vi "LSMcontroller_v65_updatedsealtest.vi"() -> ()   [LabVIEW 2015] (continued)
                                n2111 = property on="upleft" class="Bool (strict)"("Value"=w5072) -> ()  [unwired: 2 in, 2 out]
                                n2112 = property on="upright" class="Bool (strict)"("Value"=w5072) -> ()  [unwired: 2 in, 2 out]
                                n2113 = property on="downleft" class="Bool (strict)"("Value"=w5072) -> ()  [unwired: 2 in, 2 out]
                                n2114 = property on="downright" class="Bool (strict)"("Value"=w5072) -> ()  [unwired: 2 in, 2 out]
                                }
                                }
                                }
                                }
                                }
                              }
                              n2115 = dll-call lib="phlib.dll" fn="_PH_GetCountRate@8" label="PH_GetCountRate"("devidx"=w5019, "channel"=1) -> (→"Ch1Rate":i32)  [unwired: 5 in, 2 out]
                              n2116 = local read "Stop"() -> (w5021:bool)
                              n2117 = local write "points recorded"(w5018) -> ()
                            }
                          }
                          frame #3 {
                            w5081 = FALSE ("Value (Signaling)")
                            n2118 = call "2pparameters.vi"("command"="get") -> ("params out"=w5075:T10)  [unwired: 1 in]
                            n2119 = Unbundle By Name(w5075) -> ("autoshutter"=w5076:bool)
                            n2120 = case shown="True" w5076 {
                              frame False {
                              }
                              frame True {
                                n2121 = call "shuttercontrol.vi"("command"="close") -> ()  [unwired: 1 in, 1 out]
                              }
                            }
                            n2122 = property on="Start" class="Bool (strict)"("Val(Sgnl)"=w5081) -> ()  [unwired: 2 in, 2 out]
                            n2123 = property on="Start" class="Bool (strict)"("Visible"=TRUE, "DisabledEnum"=T7."Enabled" ("Disabled")) -> ()  [unwired: 2 in, 2 out]
                            n2124 = property on="Stop" class="Bool (strict)"("Val(Sgnl)"=w5081) -> ()  [unwired: 2 in, 2 out]
                            n2125 = property on="Stop" class="Bool (strict)"("Visible"=FALSE, "DisabledEnum"=T7."Disabled" ("Disabled")) -> ()  [unwired: 2 in, 2 out]
                          }
                        }
                      }
                      frame Enabled {
                      }
                    }
                    n2126 = local write "64bit disabled"(TRUE ("64bit disabled")) -> ()
                  }
                }
              }
            }
          }
          event "avpp", "Angle ref", "xpixels ref", "Vx-min ref", "Vx-max ref", "ypixels ref", "Vy-min ref", "Vy-max ref", "ROI Type", "Sampling rate": Value Change {
            n2127 = event-data() -> ()  [unwired: 1 in, 6 out]
            n2128 = local read "avpp"() -> (w5100:i32)
            n2129 = local read "Angle ref"() -> (w5099:dbl)
            n2130 = local read "ROI Type"() -> (w5098:u16)
            n2131 = local read "xpixels ref"() -> (w5095:i32)
            n2132 = local read "Vx-min ref"() -> (w5094:dbl)
            n2133 = local read "Vx-max ref"() -> (w5093:dbl)
            n2134 = local read "ypixels ref"() -> (w5091:i32)
            n2135 = local read "Vy-min ref"() -> (w5092:dbl)
            n2136 = local read "Vy-max ref"() -> (w5088:dbl)
            n2137 = local read "Sampling rate"() -> (w5083:dbl)
            n2138 = local read "# of frames"() -> (w5087:i32)
            n2139 = local read "maxbufferAI"() -> (w5086:i32)
            n2140 = local read "Override AI buffer"() -> (w5084:bool)
            n2141 = call "2pparameters.vi"("command"="get") -> ("params out"=w5097:T10)  [unwired: 1 in]
            n2142 = Bundle By Name(cluster=w5097, "avpp"=w5100, "Angle Img"=w5099, "Xpixels Img"=w5095, "Vx-min Img"=w5094, "VX-max Img"=w5093, "Ypixels Img"=w5091, "Vy-min Img"=w5092, "Vy-max Img"=w5088, "srate"=w5083, "srate Img"=w5083, "measpoints"=w5087, "maxbufferAI"=w5086, "Drawing Mode"=w5098, "Vz-reset"=0.0, "AIoverride"=w5084) -> (w5089:T10)
            n2143 = call "2pparameters.vi"("Params in"=w5089, "command"="set") -> ()  [unwired: 1 out]
          }
          event "# of frames": Value Change {
            n2144 = event-data() -> ()  [unwired: 1 in, 6 out]
            n2145 = local read "Meastab"() -> (w5101:enum32{"X-Y Image", "Linescan", "Timetrace"})
            n2146 = case shown="\"X-Y Image\", Default" w5101 {
              frame "X-Y Image", Default {
                n2147 = local read "# of frames"() -> (w5102:i32)
                n2148 = call "2pparameters.vi"("command"="get") -> ("params out"=w5106:T10)  [unwired: 1 in]
                n2149 = Bundle By Name(cluster=w5106, "measpoints"=w5102) -> (w5103:T10)
                n2150 = call "2pparameters.vi"("Params in"=w5103, "command"="set") -> ()  [unwired: 1 out]
              }
              frame "Linescan" {
                n2151 = local read "srateAODOtt"() -> (w5116:dbl)
                n2152 = local read "# of frames"() -> (w5112:i32)
                n2153 = local read "refreshtime"() -> (w5118:dbl)
                n2154 = local read "bin"() -> (w5113:dbl)
                n2155 = call "tt_timeandsamples.vi"("bin"=w5113, "refreshtime"=w5118, "srateAODOtt"=w5116, "tot#ofsamples"=w5112) -> ("refreshrate"=w5115:dbl, "refreshbuffer"=w5114:i32, "timetracecycles"=w5111:i32)  [unwired: 5 in]
                n2156 = call "2pparameters.vi"("command"="get") -> ("params out"=w5108:T10)  [unwired: 1 in]
                n2157 = Bundle By Name(cluster=w5108, "measpoints"=w5112, "tt_cycles"=w5111, "refreshbuffer"=w5114, "refreshrate"=w5115) -> (w5110:T10)
                n2158 = Reciprocal(x=w5115) -> (1/x=w5117:dbl)
                n2159 = local write "refreshtime"(w5117) -> ()
                n2160 = call "2pparameters.vi"("Params in"=w5110, "command"="set") -> ()  [unwired: 1 out]
              }
              frame "Timetrace" {
                n2161 = local read "srateAODOtt"() -> (w5128:dbl)
                n2162 = local read "# of frames"() -> (w5124:i32)
                n2163 = local read "refreshtime"() -> (w5130:dbl)
                n2164 = local read "bin"() -> (w5125:dbl)
                n2165 = call "tt_timeandsamples.vi"("bin"=w5125, "refreshtime"=w5130, "srateAODOtt"=w5128, "tot#ofsamples"=w5124) -> ("refreshrate"=w5127:dbl, "refreshbuffer"=w5126:i32, "timetracecycles"=w5123:i32)  [unwired: 5 in]
                n2166 = call "2pparameters.vi"("command"="get") -> ("params out"=w5120:T10)  [unwired: 1 in]
                n2167 = Bundle By Name(cluster=w5120, "measpoints"=w5124, "tt_cycles"=w5123, "refreshbuffer"=w5126, "refreshrate"=w5127) -> (w5122:T10)
                n2168 = Reciprocal(x=w5127) -> (1/x=w5129:dbl)
                n2169 = local write "refreshtime"(w5129) -> ()
                n2170 = call "2pparameters.vi"("Params in"=w5122, "command"="set") -> ()  [unwired: 1 out]
              }
            }
          }
          event "srateAODOtt", "refreshtime", "Vx-ref", "Vy-ref", "Vx-min draw", "Vx-max draw", "Vy-min draw", "Vy-max draw", "bin": Value Change {
            n2171 = event-data() -> ()  [unwired: 1 in, 6 out]
            n2172 = local read "ypixels ref"() -> (w5162:i32)
            n2173 = local read "Vy-min draw"() -> (w5138:dbl)
            n2174 = local read "Vy-max draw"() -> (w5137:dbl)
            n2175 = local read "Vx-min draw"() -> (w5140:dbl)
            n2176 = local read "Vx-max draw"() -> (w5139:dbl)
            n2177 = local read "xpixels ref"() -> (w5136:i32)
            n2178 = local read "ROI Type"() -> (w5135:u16)
            n2179 = local read "Pel"() -> (w5134:dbl)
            n2180 = local read "srateAODOtt"() -> (w5144:dbl)
            n2181 = local read "# of frames"() -> (w5149:i32)
            n2182 = local read "refreshtime"() -> (w5142:dbl)
            n2183 = local read "bin"() -> (w5147:dbl)
            n2184 = local read "Override AI buffer"() -> (w5132:bool)
            n2185 = local read "finite samples"() -> (w5156:bool)
            n2186 = local read "srateAODOtt"() -> (w5131:dbl)
            n2187 = local read "srateAODOtt"() -> (w5150:dbl)
            n2188 = local read "continuous"() -> (w5155:bool)
            n2189 = local read "Angle ref"() -> (w5141:dbl)
            n2190 = local read "wavdet"() -> (w5157:bool)
            n2191 = local read "Vx-ref"() -> (w5152:dbl)
            n2192 = local read "Vy-ref"() -> (w5154:dbl)
            n2193 = local read "avpp"() -> (w5153:i32)
            n2194 = call "tt_timeandsamples.vi"("bin"=w5147, "refreshtime"=w5142, "srateAODOtt"=w5144, "tot#ofsamples"=w5149) -> ("refreshrate"=w5145:dbl, "refreshbuffer"=w5146:i32, "timetracecycles"=w5151:i32)  [unwired: 5 in]
            n2195 = local read "bin"() -> (w5148:dbl)
            n2196 = call "2pparameters.vi"("command"="get") -> ("params out"=w5160:T10)  [unwired: 1 in]
            n2197 = Bundle By Name(cluster=w5160, "Drawing Mode"=w5135, "measpoints"=w5149, "tt_cycles"=w5151, "refreshbuffer"=w5146, "refreshrate"=w5145, "Vx-ref"=w5152, "Vy-ref"=w5154, "srate"=w5131, "finite"=w5156, "cont"=w5155, "wavdet"=w5157, "avpp"=w5153, "srateAODO"=w5150, "bufferAI"=w5146, "bin"=w5148, "Angle Img"=w5141, "Vxminref"=w5140, "Vxmaxref"=w5139, "Vyminref"=w5138, "Vymaxref"=w5137, "Xpixels Img"=w5136, "Ypixels Img"=w5162, "Pel"=w5134, "Vz-reset"=0.0, "AIoverride"=w5132) -> (w5158:T10)
            n2198 = Reciprocal(x=w5145) -> (1/x=w5143:dbl)
            n2199 = local write "refreshtime"(w5143) -> ()
            n2200 = call "2pparameters.vi"("Params in"=w5158, "command"="set") -> ()  [unwired: 1 out]
          }
          event "Init": Value Change {
            # "Disabled for conversion to 64 bit"
            n2201 = event-data() -> ()  [unwired: 1 in, 6 out]
            n2202 = disable-structure shown="Disabled" {
              frame Disabled {
                n2203 = flat-sequence {
                  frame #0 {
                    n2204 = local read "Measurement"() -> (w5164:T4)
                    n2205 = case shown="\"Lifetime (scan)\", \"Lifetime (contour)\"" w5164 {
                      frame "X-Y-t movie", Default {
                      }
                      frame "Lifetime (point)" {
                        n2206 = stacked-sequence {
                          frame #0 {
                            n2207 = call "initialize.vi"("mode"=0) -> ()
                          }
                          frame #1 {
                            n2208 = call "calib.vi"() -> ()  [unwired: 1 in]
                          }
                        }
                      }
                      frame "Lifetime (scan)", "Lifetime (contour)" {
                        n2209 = stacked-sequence {
                          frame #0 {
                            n2210 = call "initialize.vi"("mode"=3) -> ()
                          }
                          frame #1 {
                            n2211 = call "calib.vi"() -> ()  [unwired: 1 in]
                          }
                        }
                      }
                    }
                  }
                  frame #1 {
                    n2212 = property on="Start" class="Bool (strict)"("Visible"=TRUE, "DisabledEnum"=T7."Enabled" ("Disabled")) -> ()  [unwired: 2 in, 2 out]
                    n2213 = property on="Init" class="Bool (strict)"("Visible"=FALSE, "DisabledEnum"=T7."Disabled and Grayed Out" ("Disabled"), "Value"=FALSE ("Init")) -> ()  [unwired: 2 in, 2 out]
                  }
                }
              }
              frame Enabled {
              }
            }
            n2214 = local write "64bit disabled"(TRUE ("64bit disabled")) -> ()
          }
          event "Measurement": Value Change {
            n2215 = event-data() -> ()  [unwired: 1 in, 5 out]
            n2216 = case shown="\"Lifetime (scan)\"" "Measurement" {
              frame "X-Y-t movie" {
                w5179 = T7."Disabled" ("Disabled")
                w5178 = FALSE ("Visible")
                n2217 = call "2pparameters.vi"("command"="get") -> ("params out"=w5189:T10)  [unwired: 1 in]
                n2218 = local write "graphtab"(T5."image" ("graphtab")) -> ()
                n2219 = local write "Save tab"(enum32{"withsave", "withoutsave"}."withsave" ("Save tab")) -> ()
                n2220 = Bundle By Name(cluster=w5189, "type"="X-Y-t movie") -> (w5187:T10)
                n2221 = call "2pparameters.vi"("Params in"=w5187, "command"="set") -> ()  [unwired: 1 out]
                n2222 = property on="refreshtime" class="DigNum (strict)"("Visible"=FALSE, "DisabledEnum"=T7."Disabled and Grayed Out" ("Disabled")) -> ()  [unwired: 2 in, 2 out]
                n2223 = property on="Start" class="Bool (strict)"("Visible"=TRUE, "DisabledEnum"=T7."Enabled" ("Disabled")) -> ()  [unwired: 2 in, 2 out]
                n2224 = property on="Init" class="Bool (strict)"("Visible"=FALSE, "DisabledEnum"=T7."Disabled and Grayed Out" ("Disabled"), "Value"=FALSE ("Init")) -> ()  [unwired: 2 in, 2 out]
                n2225 = property on="ttt" class="Enum (strict)"("Visible"=FALSE) -> ()  [unwired: 2 in, 2 out]
                n2226 = property on="# of frames" class="DigNum (strict)"("DisabledEnum"=T7."Enabled" ("Disabled"), "Caption.Text"="# of frames") -> ()  [unwired: 2 in, 2 out]
                n2227 = property on="continuous" class="Bool (strict)"("Visible"=TRUE, "DisabledEnum"=T7."Enabled" ("Disabled")) -> ()  [unwired: 2 in, 2 out]
                n2228 = property on="finite samples" class="Bool (strict)"("Visible"=TRUE, "DisabledEnum"=T7."Enabled" ("Disabled")) -> ()  [unwired: 2 in, 2 out]
                n2229 = property on="avpp" class="DigNum (strict)"("Visible"=TRUE, "DisabledEnum"=T7."Enabled" ("Disabled")) -> ()  [unwired: 2 in, 2 out]
                n2230 = property on="srateAODOtt" class="DigNum (strict)"("Visible"=FALSE, "DisabledEnum"=T7."Disabled" ("Disabled")) -> ()  [unwired: 2 in, 2 out]
                n2231 = local write "save\ndata"(TRUE ("save\ndata")) -> ()
                n2232 = property on="finite samples" class="Bool (strict)"("Val(Sgnl)"=TRUE ("continuous for display")) -> ()  [unwired: 2 in, 2 out]
                n2233 = property on="continuous" class="Bool (strict)"("Value"=FALSE ("continuous for display")) -> ()  [unwired: 2 in, 2 out]
                n2234 = property on="Current Average" class="DigNum (strict)"("Visible"=TRUE, "DisabledEnum"=T7."Enabled" ("Disabled")) -> ()  [unwired: 2 in, 2 out]
                n2235 = property on="img_CH1" class="IntGraph (strict)"("ZScale.Maximum"=7.0 ("Z Scale.Range:Maximum")) -> ()  [unwired: 2 in, 2 out]
                n2236 = property on="Sampling rate" class="DigNum (strict)"("Visible"=TRUE, "DisabledEnum"=T7."Enabled" ("Disabled")) -> ()  [unwired: 2 in, 2 out]
                n2237 = property on="Pel" class="DigNum (strict)"("Visible"=w5178, "DisabledEnum"=w5179) -> ()  [unwired: 2 in, 2 out]
                n2238 = property on="bin" class="DigNum (strict)"("Visible"=w5178, "DisabledEnum"=w5179) -> ()  [unwired: 2 in, 2 out]
                "Meastab" <- enum32{"X-Y Image", "Linescan", "Timetrace"}."X-Y Image" ("Meastab")
                "Zscantab" <- enum32{"withzscan", "withoutzscan", "lifetime"}."withoutzscan" ("Zscantab")
              }
              frame "X-Y-Z stack" {
                w5216 = T7."Disabled" ("Disabled")
                w5215 = FALSE ("Visible")
                n2239 = call "2pparameters.vi"("command"="get") -> ("params out"=w5226:T10)  [unwired: 1 in]
                n2240 = call "2pparameters.vi"("command"="get") -> ("params out"=w5230:T10)  [unwired: 1 in]
                n2241 = Bundle By Name(cluster=w5226, "type"="X-Y-Z stack") -> (w5224:T10)
                n2242 = Unbundle By Name(w5230) -> ("motorref"=w5229:refnum<k7>)
                n2243 = call "2pparameters.vi"("Params in"=w5224, "command"="set") -> ()  [unwired: 1 out]
                n2244 = local write "Zscantab"(enum32{"withzscan", "withoutzscan", "lifetime"}."withzscan" ("Zscantab")) -> ()
                n2245 = local write "Meastab"(enum32{"X-Y Image", "Linescan", "Timetrace"}."X-Y Image" ("Meastab")) -> ()
                n2246 = invoke class="MG17Motor" method="GetPosition"(reference=w5229, "lChanID"=0, "pfPosition"=sgl 0.0) -> ("pfPosition"=w5241:sgl)  [unwired: 2 in, 4 out]
                n2247 = property on="refreshtime" class="DigNum (strict)"("Visible"=FALSE, "DisabledEnum"=T7."Disabled and Grayed Out" ("Disabled")) -> ()  [unwired: 2 in, 2 out]
                n2248 = property on="Start" class="Bool (strict)"("Visible"=TRUE, "DisabledEnum"=T7."Enabled" ("Disabled")) -> ()  [unwired: 2 in, 2 out]
                n2249 = property on="Init" class="Bool (strict)"("Visible"=FALSE, "DisabledEnum"=T7."Disabled and Grayed Out" ("Disabled"), "Value"=FALSE ("Init")) -> ()  [unwired: 2 in, 2 out]
                n2250 = property on="ttt" class="Enum (strict)"("Visible"=FALSE) -> ()  [unwired: 2 in, 2 out]
                n2251 = Multiply(x=w5241, y=1000.0) -> (x*y=w5240:dbl)
                n2252 = local write "Actual Z position"(w5240) -> ()
                n2253 = local write "Save tab"(enum32{"withsave", "withoutsave"}."withsave" ("Save tab")) -> ()
                n2254 = property on="finite samples" class="Bool (strict)"("Visible"=FALSE, "DisabledEnum"=T7."Disabled and Grayed Out" ("Disabled")) -> ()  [unwired: 2 in, 2 out]
                n2255 = property on="avpp" class="DigNum (strict)"("Visible"=TRUE, "DisabledEnum"=T7."Enabled" ("Disabled")) -> ()  [unwired: 2 in, 2 out]
                n2256 = property on="continuous" class="Bool (strict)"("Visible"=FALSE, "DisabledEnum"=T7."Disabled and Grayed Out" ("Disabled")) -> ()  [unwired: 2 in, 2 out]
                n2257 = property on="img_CH1" class="IntGraph (strict)"("ZScale.Maximum"=7.0 ("Z Scale.Range:Maximum")) -> ()  [unwired: 2 in, 2 out]
                n2258 = property on="srateAODOtt" class="DigNum (strict)"("Visible"=FALSE, "DisabledEnum"=T7."Disabled" ("Disabled")) -> ()  [unwired: 2 in, 2 out]
                n2259 = property on="Pel" class="DigNum (strict)"("Visible"=w5215, "DisabledEnum"=w5216) -> ()  [unwired: 2 in, 2 out]
                n2260 = property on="bin" class="DigNum (strict)"("Visible"=w5215, "DisabledEnum"=w5216) -> ()  [unwired: 2 in, 2 out]
                n2261 = property on="Current Average" class="DigNum (strict)"("Visible"=TRUE, "DisabledEnum"=T7."Enabled" ("Disabled")) -> ()  [unwired: 2 in, 2 out]
                n2262 = property on="# of frames" class="DigNum (strict)"("Caption.Text"="# of slices", "DisabledEnum"=T7."Disabled and Grayed Out" ("Disabled")) -> ()  [unwired: 2 in, 2 out]
                n2263 = local write "save\ndata"(TRUE ("save\ndata")) -> ()
                n2264 = property on="finite samples" class="Bool (strict)"("Val(Sgnl)"=TRUE ("continuous for display")) -> ()  [unwired: 2 in, 2 out]
                n2265 = property on="continuous" class="Bool (strict)"("Value"=FALSE ("continuous for display")) -> ()  [unwired: 2 in, 2 out]
                n2266 = property on="Sampling rate" class="DigNum (strict)"("Visible"=TRUE, "DisabledEnum"=T7."Enabled" ("Disabled")) -> ()  [unwired: 2 in, 2 out]
              }
              frame "X-Y-Z-t movie" {
                w5260 = T7."Disabled" ("Disabled")
                w5259 = FALSE ("Visible")
                n2267 = property on="# of frames" class="DigNum (strict)"("DisabledEnum"=T7."Enabled" ("Disabled")) -> ()  [unwired: 2 in, 2 out]
                n2268 = property on="Current Average" class="DigNum (strict)"("Visible"=TRUE, "DisabledEnum"=T7."Enabled" ("Disabled")) -> ()  [unwired: 2 in, 2 out]
                n2269 = property on="avpp" class="DigNum (strict)"("Visible"=TRUE, "DisabledEnum"=T7."Enabled" ("Disabled")) -> ()  [unwired: 2 in, 2 out]
                n2270 = local write "Save tab"(enum32{"withsave", "withoutsave"}."withsave" ("Save tab")) -> ()
                n2271 = local write "Zscantab"(enum32{"withzscan", "withoutzscan", "lifetime"}."withzscan" ("Zscantab")) -> ()
                n2272 = local write "Meastab"(enum32{"X-Y Image", "Linescan", "Timetrace"}."X-Y Image" ("Meastab")) -> ()
                n2273 = property on="Start" class="Bool (strict)"("Visible"=TRUE, "DisabledEnum"=T7."Enabled" ("Disabled")) -> ()  [unwired: 2 in, 2 out]
                n2274 = property on="refreshtime" class="DigNum (strict)"("Visible"=FALSE, "DisabledEnum"=T7."Disabled and Grayed Out" ("Disabled")) -> ()  [unwired: 2 in, 2 out]
                n2275 = property on="Init" class="Bool (strict)"("Visible"=FALSE, "DisabledEnum"=T7."Disabled and Grayed Out" ("Disabled"), "Value"=FALSE ("Init")) -> ()  [unwired: 2 in, 2 out]
                n2276 = property on="ttt" class="Enum (strict)"("Visible"=FALSE) -> ()  [unwired: 2 in, 2 out]
                n2277 = call "2pparameters.vi"("command"="get") -> ("params out"=w5270:T10)  [unwired: 1 in]
                n2278 = Bundle By Name(cluster=w5270, "type"="X-Y-Z-t movie") -> (w5268:T10)
                n2279 = property on="continuous" class="Bool (strict)"("Visible"=TRUE, "DisabledEnum"=T7."Enabled" ("Disabled")) -> ()  [unwired: 2 in, 2 out]
                n2280 = property on="finite samples" class="Bool (strict)"("Visible"=TRUE, "DisabledEnum"=T7."Enabled" ("Disabled")) -> ()  [unwired: 2 in, 2 out]
                n2281 = call "2pparameters.vi"("Params in"=w5268, "command"="set") -> ()  [unwired: 1 out]
                n2282 = property on="srateAODOtt" class="DigNum (strict)"("Visible"=FALSE, "DisabledEnum"=T7."Disabled" ("Disabled")) -> ()  [unwired: 2 in, 2 out]
                n2283 = local write "save\ndata"(TRUE ("save\ndata")) -> ()
                n2284 = property on="img_CH1" class="IntGraph (strict)"("ZScale.Maximum"=7.0 ("Z Scale.Range:Maximum")) -> ()  [unwired: 2 in, 2 out]
                n2285 = property on="continuous" class="Bool (strict)"("Value"=FALSE ("continuous for display")) -> ()  [unwired: 2 in, 2 out]
                n2286 = property on="finite samples" class="Bool (strict)"("Value"=TRUE ("continuous for display")) -> ()  [unwired: 2 in, 2 out]
                n2287 = property on="Sampling rate" class="DigNum (strict)"("Visible"=TRUE, "DisabledEnum"=T7."Enabled" ("Disabled")) -> ()  [unwired: 2 in, 2 out]
                n2288 = property on="Pel" class="DigNum (strict)"("Visible"=w5259, "DisabledEnum"=w5260) -> ()  [unwired: 2 in, 2 out]
                n2289 = property on="bin" class="DigNum (strict)"("Visible"=w5259, "DisabledEnum"=w5260) -> ()  [unwired: 2 in, 2 out]
              }
              frame "linescan" {
                w5295 = T7."Enabled" ("Disabled")
                w5294 = TRUE ("Visible")
                w5297 = T7."Enabled" ("Disabled")
                w5296 = TRUE ("Visible")
                n2290 = local write "Meastab"(enum32{"X-Y Image", "Linescan", "Timetrace"}."Linescan" ("Meastab")) -> ()
                n2291 = property on="Current Average" class="DigNum (strict)"("Visible"=TRUE, "DisabledEnum"=T7."Enabled" ("Disabled")) -> ()  [unwired: 2 in, 2 out]
                n2292 = property on="ttt" class="Enum (strict)"("Visible"=FALSE) -> ()  [unwired: 2 in, 2 out]
                n2293 = local write "Save tab"(enum32{"withsave", "withoutsave"}."withsave" ("Save tab")) -> ()
                n2294 = local write "Zscantab"(enum32{"withzscan", "withoutzscan", "lifetime"}."withoutzscan" ("Zscantab")) -> ()
                n2295 = property on="refreshtime" class="DigNum (strict)"("Visible"=FALSE, "DisabledEnum"=T7."Disabled and Grayed Out" ("Disabled")) -> ()  [unwired: 2 in, 2 out]
                n2296 = property on="continuous" class="Bool (strict)"("Value"=FALSE ("continuous for display")) -> ()  [unwired: 2 in, 2 out]
                n2297 = property on="finite samples" class="Bool (strict)"("Value"=TRUE ("continuous for display")) -> ()  [unwired: 2 in, 2 out]
                n2298 = local write "save\ndata"(TRUE ("save\ndata")) -> ()
                n2299 = property on="Start" class="Bool (strict)"("Visible"=TRUE, "DisabledEnum"=T7."Enabled" ("Disabled")) -> ()  [unwired: 2 in, 2 out]
                n2300 = property on="Init" class="Bool (strict)"("Visible"=FALSE, "DisabledEnum"=T7."Disabled and Grayed Out" ("Disabled"), "Value"=FALSE ("Init")) -> ()  [unwired: 2 in, 2 out]
                n2301 = call "2pparameters.vi"("command"="get") -> ("params out"=w5306:T10)  [unwired: 1 in]
                n2302 = Bundle By Name(cluster=w5306, "type"="linescan") -> (w5304:T10)
                n2303 = property on="# of frames" class="DigNum (strict)"("DisabledEnum"=T7."Enabled" ("Disabled"), "Caption.Text"="# of lines") -> ()  [unwired: 2 in, 2 out]
                n2304 = property on="continuous" class="Bool (strict)"("Visible"=TRUE, "DisabledEnum"=T7."Enabled" ("Disabled")) -> ()  [unwired: 2 in, 2 out]
                n2305 = property on="avpp" class="DigNum (strict)"("Visible"=TRUE, "DisabledEnum"=T7."Enabled" ("Disabled")) -> ()  [unwired: 2 in, 2 out]
                n2306 = property on="finite samples" class="Bool (strict)"("Visible"=TRUE, "DisabledEnum"=T7."Enabled" ("Disabled")) -> ()  [unwired: 2 in, 2 out]
                n2307 = property on="srateAODOtt" class="DigNum (strict)"("Visible"=TRUE, "DisabledEnum"=T7."Enabled" ("Disabled")) -> ()  [unwired: 2 in, 2 out]
                n2308 = call "2pparameters.vi"("Params in"=w5304, "command"="set") -> ()  [unwired: 1 out]
                n2309 = property on="Pel" class="DigNum (strict)"("Visible"=w5296, "DisabledEnum"=w5297) -> ()  [unwired: 2 in, 2 out]
                n2310 = property on="bin" class="DigNum (strict)"("Visible"=w5296, "DisabledEnum"=w5297) -> ()  [unwired: 2 in, 2 out]
                n2311 = property on="Sampling rate" class="DigNum (strict)"("Visible"=FALSE, "DisabledEnum"=T7."Disabled" ("Disabled")) -> ()  [unwired: 2 in, 2 out]
                n2312 = property on="Pel" class="DigNum (strict)"("Visible"=w5294, "DisabledEnum"=w5295) -> ()  [unwired: 2 in, 2 out]
                n2313 = property on="bin" class="DigNum (strict)"("Visible"=w5294, "DisabledEnum"=w5295) -> ()  [unwired: 2 in, 2 out]
              }
              frame "Timetrace" {
                w5332 = T7."Enabled" ("Disabled")
                w5331 = TRUE ("Visible")
                n2314 = call "2pparameters.vi"("command"="get") -> ("params out"=w5337:T10)  [unwired: 1 in]
                n2315 = local write "Meastab"(enum32{"X-Y Image", "Linescan", "Timetrace"}."Timetrace" ("Meastab")) -> ()
                n2316 = Unbundle By Name(w5337) -> ("Angle draw"=w5339:dbl)
                n2317 = local write "Zscantab"(enum32{"withzscan", "withoutzscan", "lifetime"}."withoutzscan" ("Zscantab")) -> ()
                n2318 = property on="# of frames" class="DigNum (strict)"("DisabledEnum"=T7."Enabled" ("Disabled"), "Caption.Text"="# of samples") -> ()  [unwired: 2 in, 2 out]
                n2319 = property on="refreshtime" class="DigNum (strict)"("Visible"=TRUE, "DisabledEnum"=T7."Enabled" ("Disabled")) -> ()  [unwired: 2 in, 2 out]
                n2320 = property on="avpp" class="DigNum (strict)"("Visible"=FALSE, "DisabledEnum"=T7."Disabled and Grayed Out" ("Disabled")) -> ()  [unwired: 2 in, 2 out]
                n2321 = property on="Current Average" class="DigNum (strict)"("Visible"=FALSE, "DisabledEnum"=T7."Disabled and Grayed Out" ("Disabled")) -> ()  [unwired: 2 in, 2 out]
                n2322 = local write "Angle drawing"(w5339) -> ()
                n2323 = property on="ttt" class="Enum (strict)"("Visible"=TRUE) -> ()  [unwired: 2 in, 2 out]
                n2324 = property on="continuous" class="Bool (strict)"("Visible"=TRUE, "DisabledEnum"=T7."Enabled" ("Disabled")) -> ()  [unwired: 2 in, 2 out]
                n2325 = property on="finite samples" class="Bool (strict)"("Visible"=TRUE, "DisabledEnum"=T7."Enabled" ("Disabled")) -> ()  [unwired: 2 in, 2 out]
                n2326 = local write "save\ndata"(TRUE ("save\ndata")) -> ()
                n2327 = property on="finite samples" class="Bool (strict)"("Val(Sgnl)"=TRUE ("continuous for display")) -> ()  [unwired: 2 in, 2 out]
                n2328 = property on="continuous" class="Bool (strict)"("Value"=FALSE ("continuous for display")) -> ()  [unwired: 2 in, 2 out]
                n2329 = local write "Save tab"(enum32{"withsave", "withoutsave"}."withsave" ("Save tab")) -> ()
                n2330 = property on="srateAODOtt" class="DigNum (strict)"("Visible"=TRUE, "DisabledEnum"=T7."Enabled" ("Disabled")) -> ()  [unwired: 2 in, 2 out]
                n2331 = call "2pparameters.vi"("command"="get") -> ("params out"=w5344:T10)  [unwired: 1 in]
                n2332 = property on="Start" class="Bool (strict)"("Visible"=TRUE, "DisabledEnum"=T7."Enabled" ("Disabled")) -> ()  [unwired: 2 in, 2 out]
                n2333 = property on="Init" class="Bool (strict)"("Visible"=FALSE, "DisabledEnum"=T7."Disabled and Grayed Out" ("Disabled"), "Value"=FALSE ("Init")) -> ()  [unwired: 2 in, 2 out]
                n2334 = Bundle By Name(cluster=w5344, "type"="Timetrace") -> (w5342:T10)
                n2335 = property on="Sampling rate" class="DigNum (strict)"("Visible"=FALSE, "DisabledEnum"=T7."Disabled" ("Disabled")) -> ()  [unwired: 2 in, 2 out]
                n2336 = property on="Pel" class="DigNum (strict)"("Visible"=w5331, "DisabledEnum"=w5332) -> ()  [unwired: 2 in, 2 out]
                n2337 = property on="bin" class="DigNum (strict)"("Visible"=w5331, "DisabledEnum"=w5332) -> ()  [unwired: 2 in, 2 out]
                n2338 = call "2pparameters.vi"("Params in"=w5342, "command"="set") -> ()  [unwired: 1 out]
              }
              frame "Lifetime (point)" {
                w5365 = T7."Enabled" ("Disabled")
                w5364 = TRUE ("Visible")
                n2339 = property on="Pel" class="DigNum (strict)"("Visible"=w5364, "DisabledEnum"=w5365) -> ()  [unwired: 2 in, 2 out]
                n2340 = property on="bin" class="DigNum (strict)"("Visible"=w5364, "DisabledEnum"=w5365) -> ()  [unwired: 2 in, 2 out]
                n2341 = property on="ttt" class="Enum (strict)"("Visible"=FALSE) -> ()  [unwired: 2 in, 2 out]
                n2342 = local write "Zscantab"(enum32{"withzscan", "withoutzscan", "lifetime"}."lifetime" ("Zscantab")) -> ()
                n2343 = local write "graphtab"(T5."Lifetime" ("graphtab")) -> ()
                n2344 = local write "Meastab"(enum32{"X-Y Image", "Linescan", "Timetrace"}."Timetrace" ("Meastab")) -> ()
                n2345 = call "lifetimeparameters.vi"("command"="get") -> ("Params out"=w5372:T19)  [unwired: 1 in]
                n2346 = Unbundle By Name(w5372) -> ("initialized"=w5373:bool)
                n2347 = property on="srateAODOtt" class="DigNum (strict)"("Visible"=TRUE, "DisabledEnum"=T7."Enabled" ("Disabled")) -> ()  [unwired: 2 in, 2 out]
                n2348 = case shown="False" w5373 {
                  frame False {
                    n2349 = property on="Init" class="Bool (strict)"("Visible"=TRUE, "DisabledEnum"=T7."Enabled" ("Disabled")) -> ()  [unwired: 2 in, 2 out]
                    n2350 = property on="Start" class="Bool (strict)"("Visible"=FALSE, "DisabledEnum"=T7."Disabled and Grayed Out" ("Disabled")) -> ()  [unwired: 2 in, 2 out]
                  }
                  frame True {
                  }
                }
                n2351 = property on="Sampling rate" class="DigNum (strict)"("Visible"=FALSE, "DisabledEnum"=T7."Disabled" ("Disabled")) -> ()  [unwired: 2 in, 2 out]
              }
              frame "Lifetime (scan)" {
                w5382 = T7."Disabled" ("Disabled")
                w5381 = FALSE ("Visible")
                n2352 = call "lifetimeparameters.vi"("command"="get") -> ("Params out"=w5394:T19)  [unwired: 1 in]
                n2353 = local write "graphtab"(T5."image" ("graphtab")) -> ()
                n2354 = local write "Save tab"(enum32{"withsave", "withoutsave"}."withsave" ("Save tab")) -> ()
                n2355 = local write "Meastab"(enum32{"X-Y Image", "Linescan", "Timetrace"}."X-Y Image" ("Meastab")) -> ()
                n2356 = local write "Zscantab"(enum32{"withzscan", "withoutzscan", "lifetime"}."lifetime" ("Zscantab")) -> ()
                n2357 = Unbundle By Name(w5394) -> ("initialized"=w5393:bool)
                n2358 = property on="ttt" class="Enum (strict)"("Visible"=FALSE) -> ()  [unwired: 2 in, 2 out]
                n2359 = property on="refreshtime" class="DigNum (strict)"("Visible"=FALSE, "DisabledEnum"=T7."Disabled and Grayed Out" ("Disabled")) -> ()  [unwired: 2 in, 2 out]
                n2360 = property on="Pel" class="DigNum (strict)"("Visible"=w5381, "DisabledEnum"=w5382) -> ()  [unwired: 2 in, 2 out]
                n2361 = property on="bin" class="DigNum (strict)"("Visible"=w5381, "DisabledEnum"=w5382) -> ()  [unwired: 2 in, 2 out]
                n2362 = property on="save data" class="Bool (strict)"("Visible"=TRUE, "DisabledEnum"=T7."Enabled" ("Disabled"), "Value"=TRUE ("Visible")) -> ()  [unwired: 2 in, 2 out]
                n2363 = case shown="False" w5393 {
                  frame False {
                    n2364 = property on="Init" class="Bool (strict)"("Visible"=TRUE, "DisabledEnum"=T7."Enabled" ("Disabled")) -> ()  [unwired: 2 in, 2 out]
                    n2365 = property on="Start" class="Bool (strict)"("Visible"=FALSE, "DisabledEnum"=T7."Disabled and Grayed Out" ("Disabled")) -> ()  [unwired: 2 in, 2 out]
                  }
                  frame True {
                  }
                }
                n2366 = call "2pparameters.vi"("command"="get") -> ("params out"=w5399:T10)  [unwired: 1 in]
                n2367 = property on="continuous" class="Bool (strict)"("Visible"=TRUE, "DisabledEnum"=T7."Disabled and Grayed Out" ("Disabled")) -> ()  [unwired: 2 in, 2 out]
                n2368 = property on="finite samples" class="Bool (strict)"("Visible"=TRUE, "DisabledEnum"=T7."Enabled" ("Disabled")) -> ()  [unwired: 2 in, 2 out]
                n2369 = Bundle By Name(cluster=w5399, "type"="Lifetime (scan)") -> (w5397:T10)
                n2370 = call "2pparameters.vi"("Params in"=w5397, "command"="set") -> ()  [unwired: 1 out]
                n2371 = property on="finite samples" class="Bool (strict)"("Val(Sgnl)"=TRUE ("continuous for display")) -> ()  [unwired: 2 in, 2 out]
                n2372 = property on="continuous" class="Bool (strict)"("Value"=FALSE ("continuous for display")) -> ()  [unwired: 2 in, 2 out]
                n2373 = property on="srateAODOtt" class="DigNum (strict)"("Visible"=FALSE, "DisabledEnum"=T7."Disabled" ("Disabled")) -> ()  [unwired: 2 in, 2 out]
                n2374 = property on="# of frames" class="DigNum (strict)"("DisabledEnum"=T7."Enabled" ("Disabled"), "Caption.Text"="# of frames") -> ()  [unwired: 2 in, 2 out]
                n2375 = property on="img_CH1" class="IntGraph (strict)"("ZScale.Maximum"=12.5 ("Z Scale.Range:Maximum")) -> ()  [unwired: 2 in, 2 out]
                n2376 = property on="Current Average" class="DigNum (strict)"("Visible"=TRUE, "DisabledEnum"=T7."Enabled" ("Disabled")) -> ()  [unwired: 2 in, 2 out]
                n2377 = property on="Sampling rate" class="DigNum (strict)"("Visible"=TRUE, "DisabledEnum"=T7."Enabled" ("Disabled")) -> ()  [unwired: 2 in, 2 out]
                n2378 = property on="avpp" class="DigNum (strict)"("Visible"=TRUE, "DisabledEnum"=T7."Enabled" ("Disabled")) -> ()  [unwired: 2 in, 2 out]
              }
              frame "Lifetime (contour)" {
                w5423 = T7."Enabled" ("Disabled")
                w5422 = TRUE ("Visible")
                n2379 = call "2pparameters.vi"("command"="get") -> ("params out"=w5430:T10)  [unwired: 1 in]
                n2380 = property on="# of frames" class="DigNum (strict)"("DisabledEnum"=T7."Enabled" ("Disabled"), "Caption.Text"="# of samples") -> ()  [unwired: 2 in, 2 out]
                n2381 = property on="refreshtime" class="DigNum (strict)"("Visible"=TRUE, "DisabledEnum"=T7."Enabled" ("Disabled")) -> ()  [unwired: 2 in, 2 out]
                n2382 = Unbundle By Name(w5430) -> ("Angle draw"=w5432:dbl)
                n2383 = property on="avpp" class="DigNum (strict)"("Visible"=FALSE, "DisabledEnum"=T7."Disabled and Grayed Out" ("Disabled")) -> ()  [unwired: 2 in, 2 out]
                n2384 = property on="Current Average" class="DigNum (strict)"("Visible"=FALSE, "DisabledEnum"=T7."Disabled and Grayed Out" ("Disabled")) -> ()  [unwired: 2 in, 2 out]
                n2385 = local write "Angle drawing"(w5432) -> ()
                n2386 = local write "Save tab"(enum32{"withsave", "withoutsave"}."withsave" ("Save tab")) -> ()
                n2387 = local write "Zscantab"(enum32{"withzscan", "withoutzscan", "lifetime"}."lifetime" ("Zscantab")) -> ()
                n2388 = local write "graphtab"(T5."Lifetime" ("graphtab")) -> ()
                n2389 = local write "Meastab"(enum32{"X-Y Image", "Linescan", "Timetrace"}."Timetrace" ("Meastab")) -> ()
                n2390 = property on="ttt" class="Enum (strict)"("Visible"=TRUE) -> ()  [unwired: 2 in, 2 out]
                n2391 = call "lifetimeparameters.vi"("command"="get") -> ("Params out"=w5454:T19)  [unwired: 1 in]
                n2392 = property on="finite samples" class="Bool (strict)"("Val(Sgnl)"=TRUE ("continuous for display")) -> ()  [unwired: 2 in, 2 out]
                n2393 = local write "save\ndata"(TRUE ("save\ndata")) -> ()
                n2394 = Unbundle By Name(w5454) -> ("initialized"=w5455:bool)
                n2395 = property on="continuous" class="Bool (strict)"("Visible"=TRUE, "DisabledEnum"=T7."Enabled" ("Disabled")) -> ()  [unwired: 2 in, 2 out]
                n2396 = property on="finite samples" class="Bool (strict)"("Visible"=TRUE, "DisabledEnum"=T7."Enabled" ("Disabled")) -> ()  [unwired: 2 in, 2 out]
                n2397 = property on="Pel" class="DigNum (strict)"("Visible"=w5422, "DisabledEnum"=w5423) -> ()  [unwired: 2 in, 2 out]
                n2398 = property on="bin" class="DigNum (strict)"("Visible"=w5422, "DisabledEnum"=w5423) -> ()  [unwired: 2 in, 2 out]
                n2399 = property on="continuous" class="Bool (strict)"("Value"=FALSE ("continuous for display")) -> ()  [unwired: 2 in, 2 out]
                n2400 = case shown="False" w5455 {
                  frame False {
                    n2401 = property on="Init" class="Bool (strict)"("Visible"=TRUE, "DisabledEnum"=T7."Enabled" ("Disabled")) -> ()  [unwired: 2 in, 2 out]
                    n2402 = property on="Start" class="Bool (strict)"("Visible"=FALSE, "DisabledEnum"=T7."Disabled and Grayed Out" ("Disabled")) -> ()  [unwired: 2 in, 2 out]
                  }
                  frame True {
                  }
                }
                n2403 = property on="srateAODOtt" class="DigNum (strict)"("Visible"=TRUE, "DisabledEnum"=T7."Enabled" ("Disabled")) -> ()  [unwired: 2 in, 2 out]
                n2404 = call "2pparameters.vi"("command"="get") -> ("params out"=w5434:T10)  [unwired: 1 in]
                n2405 = Bundle By Name(cluster=w5434, "type"="Timetrace") -> (w5428:T10)
                n2406 = call "2pparameters.vi"("Params in"=w5428, "command"="set") -> ()  [unwired: 1 out]
                n2407 = property on="Sampling rate" class="DigNum (strict)"("Visible"=FALSE, "DisabledEnum"=T7."Disabled" ("Disabled")) -> ()  [unwired: 2 in, 2 out]
              }
            }
          }
          event "Laserpower \n(%)": Value Change {
            n2408 = event-data() -> ("OldVal"=w5463:dbl, "NewVal"=w5464:dbl)  [unwired: 1 in, 4 out]
            n2409 = Not Equal?(x=w5463, y=w5464) -> (x != y?=w5465:bool)
            n2410 = case shown="True" w5465 {
              tunnel: w5464 -> [_ w5467]
              frame False {
              }
              frame True {
                n2411 = local read "wavelength(nm)"() -> (w5468:dbl)
                n2412 = call "configuration.vi"("command"="get") -> ("config out"=w5472:T11)  [unwired: 2 in, 1 out]
                n2413 = call "pockelscellcalibration.vi"("l"=w5468, "T"=w5467) -> ("Vout"=w5466:dbl)
                n2414 = Unbundle By Name(w5472) -> ("Vto2P"=w5471:i32, "AOlines"=w5470:tag[])
                n2415 = property on="lpow" class="DigNum (strict)"("Value"=w5467) -> ()  [unwired: 2 in, 2 out]
                n2416 = local write "Vpockels"(w5466) -> ()
                n2417 = Index Array(array=w5470, index=w5471) -> (element=w5469:tag)
                n2418 = call-poly <vilib>:"DAQmx Create Virtual Channel.vi"("physical channels"=w5469) -> ("task out"=w5475:refnum<k21>, "error out"=w5474:errorcluster)  [unwired: 13 in]
                n2419 = call-poly <vilib>:"DAQmx Write.vi"("task/channels in"=w5475, "data"=w5466, "error in"=w5474) -> ("task out"=w5476:refnum<k21>, "error out"=w5477:errorcluster)  [unwired: 10 in, 1 out]
                n2420 = call <vilib>:"DAQmx Start Task.vi"("task/channels in"=w5476, "error in"=w5477) -> ("task out"=w5478:refnum<k21>, "error out"=w5479:errorcluster)  [unwired: 12 in]
                n2421 = call <vilib>:"DAQmx Stop Task.vi"("task/channels in"=w5478, "error in"=w5479) -> ("task out"=w5480:refnum<k21>, "error out"=w5481:errorcluster)  [unwired: 12 in]
                n2422 = call <vilib>:"DAQmx Clear Task.vi"("task in"=w5480, "error in"=w5481) -> ()  [unwired: 13 in, 1 out]
              }
            }
          }
          event "lpow": Value Change {
            n2423 = event-data() -> ("OldVal"=w5482:dbl, "NewVal"=w5483:dbl)  [unwired: 1 in, 4 out]
            n2424 = Not Equal?(x=w5482, y=w5483) -> (x != y?=w5484:bool)
            n2425 = case shown="True" w5484 {
              tunnel: w5483 -> [_ w5487]
              frame False {
              }
              frame True {
                n2426 = local read "wavelength(nm)"() -> (w5486:dbl)
                n2427 = call "pockelscellcalibration.vi"("l"=w5486, "T"=w5487) -> ("Vout"=w5485:dbl)
                n2428 = call "configuration.vi"("command"="get") -> ("config out"=w5491:T11)  [unwired: 2 in, 1 out]
                n2429 = Unbundle By Name(w5491) -> ("Vto2P"=w5490:i32, "AOlines"=w5489:tag[])
                n2430 = local write "Vpockels"(w5485) -> ()
                n2431 = property on="Laserpower \n(%)" class="Slide (strict)"("Value"=w5487) -> ()  [unwired: 2 in, 2 out]
                n2432 = Index Array(array=w5489, index=w5490) -> (element=w5488:tag)
                n2433 = call-poly <vilib>:"DAQmx Create Virtual Channel.vi"("physical channels"=w5488) -> ("task out"=w5494:refnum<k21>, "error out"=w5493:errorcluster)  [unwired: 13 in]
                n2434 = call-poly <vilib>:"DAQmx Write.vi"("task/channels in"=w5494, "data"=w5485, "error in"=w5493) -> ("task out"=w5495:refnum<k21>, "error out"=w5496:errorcluster)  [unwired: 10 in, 1 out]
                n2435 = call <vilib>:"DAQmx Start Task.vi"("task/channels in"=w5495, "error in"=w5496) -> ("task out"=w5497:refnum<k21>, "error out"=w5498:errorcluster)  [unwired: 12 in]
                n2436 = call <vilib>:"DAQmx Stop Task.vi"("task/channels in"=w5497, "error in"=w5498) -> ("task out"=w5499:refnum<k21>, "error out"=w5500:errorcluster)  [unwired: 12 in]
                n2437 = call <vilib>:"DAQmx Clear Task.vi"("task in"=w5499, "error in"=w5500) -> ()  [unwired: 13 in, 1 out]
              }
            }
          }
          event "sealtest": Value Change {
            n2438 = event-data() -> ()  [unwired: 1 in, 6 out]
            n2439 = case shown="True" "sealtest" {
              frame False {
              }
              frame True {
                n2440 = stacked-sequence {
                  seq-local: [w5502 _ _ _ _ _ _] -> [_ w5535 _ w5587 _ _ _]
                  frame #0 {
                    n2441 = stacked-sequence {
                      tunnel: [_ w5514 _] -> w5502
                      frame #0 {
                        n2442 = call "2pparameters.vi"("command"="get") -> ("params out"=w5507:T10)  [unwired: 1 in]
                        n2443 = Unbundle By Name(w5507) -> ("autoshutter"=w5508:bool)
                        n2444 = local read "OCchecked?"() -> (w5505:bool)
                        n2445 = call "sealtestwfparams.vi"("command"="set") -> ()  [unwired: 6 in, 1 out]
                        n2446 = case shown="False" w5505 {
                          frame False {
                            n2447 = One Button Dialog(message="Is the OC gain correct?", button name ("OK")="ok") -> (true=w5509:bool)
                            n2448 = local write "OCchecked?"(w5509) -> ()
                          }
                          frame True {
                          }
                        }
                        n2449 = case shown="True" w5508 {
                          frame False {
                          }
                          frame True {
                            n2450 = call "shuttercontrol.vi"("command"="close") -> ()  [unwired: 1 in, 1 out]
                          }
                        }
                        n2451 = call "allAI-temp.vi"("command"=enum16{"get", "set", "clear", "append"}."clear") -> ()  [unwired: 3 in, 2 out]
                      }
                      frame #1 {
                        n2452 = call "sealtestwfparams.vi"("command"="get") -> ("Params out"=w5520:T22)  [unwired: 6 in]
                        n2453 = Unbundle By Name(w5520) -> ("AO parameters"=w5518:T23)
                        n2454 = Index Array(array=w5518, index=0) -> (element=w5517:T24)
                        n2455 = call "generateRampedSquareWave_fromAOparameters.vi"("AO params"=w5517) -> ("Waveform"=w5513:waveform(dbl), "wflength"=w5514:i32)
                        n2456 = Build Array(w5513) -> (w5516:waveform(dbl)[])
                        n2457 = call "waveformssealtestbuffer.vi"("AO wf in"=w5516, "command"="set") -> ()  [unwired: 1 out]
                      }
                      frame #2 {
                        n2458 = local read "Vholding (mV)"() -> (w5523:sgl)
                        n2459 = local read "Current Clamp"() -> (w5529:bool)
                        n2460 = local read "Voltage Clamp"() -> (w5528:bool)
                        n2461 = local read "OCgain"() -> (w5524:sgl)
                        n2462 = local read "CC_ICgain"() -> (w5527:dbl)
                        n2463 = local read "holdon"() -> (w5522:bool)
                        n2464 = call "patchparameters.vi"("command"="get") -> ("Params out"=w5531:T13)  [unwired: 1 in]
                        n2465 = Bundle By Name(cluster=w5531, "VC"=w5528, "CC"=w5529, "CC_icg (pA/mv)"=w5527, "VC_icg (mV/mV)"=10.0, "OCG (mV/pA)"=w5524, "OVG (mV/mV)"=0.1, "Vhold (mV)"=w5523, "holdon"=w5522) -> (w5530:T13)
                        n2466 = call "patchparameters.vi"("Params in"=w5530, "command"="set") -> ()  [unwired: 1 out]
                      }
                    }
                  }
                  frame #1 {
                    w5534 = 2
                    n2467 = call "patchparameters.vi"("command"="get") -> ("Params out"=w5542:T13)  [unwired: 1 in]
                    n2468 = Unbundle By Name(w5542) -> ("holdon"=w5541:bool, "Vhold (mV)"=w5540:sgl, "CC_icg (pA/mv)"=w5548:sgl, "CC"=w5546:bool, "VC_icg (mV/mV)"=w5547:sgl)
                    n2469 = Select(t=w5548, s=w5546, f=w5547) -> (s? t:f=w5549:sgl)
                    n2470 = To Single Precision Float(number=0.001 ("y")) -> (single precision float=w5550:sgl)
                    n2471 = Compound Arithmetic op=MULTIPLY(w5540, w5549, w5550) -> (w5544:sgl)
                    n2472 = case shown="False" w5541 {
                      tunnel: w5544 -> [_ w5562]
                      tunnel: [0.0 w5562] -> w5537
                      frame False {
                      }
                      frame True {
                      }
                    }
                    n2473 = Greater Than 0?(x=w5534) -> (x > 0?=w5536:bool)
                    n2474 = case shown="True" w5536 {
                      tunnel: w5535 -> [_ w5551]
                      tunnel: w5534 -> [_ w5554]
                      frame False {
                      }
                      frame True {
                        n2475 = Initialize Array(sgl 0.0 ("element"), w5554, w5551) -> (w5552:sgl[][])
                        n2476 = call "allAI-temp.vi"("array in"=w5552, "command"=enum16{"get", "set", "clear", "append"}."set") -> ()  [unwired: 2 in, 2 out]
                      }
                    }
                    n2477 = flat-sequence {
                      tunnel: w5535 -> [w5558]
                      tunnel: w5535 -> [w5557]
                      tunnel: [w5557] -> w5539
                      tunnel: [w5556] -> w5538
                      tunnel: w5537 -> [w5556]
                      tunnel: w5539 -> [w5560]
                      tunnel: w5538 -> [w5559]
                      frame #0 {
                        n2478 = call "prepAI_sealtest.vi"("samples per channel"=w5558) -> ()  [unwired: 2 in]
                      }
                      frame #1 {
                        n2479 = call "prepAO_sealtest.vi"("Vhold"=w5559, "samples per channel"=w5560) -> ()  [unwired: 1 in]
                      }
                    }
                  }
                  frame #2 {
                    n2480 = stacked-sequence {
                      frame #0 {
                        n2481 = call "tempconfigAO_seal.vi"("command"="get") -> ("Temp Config out"=w5566:T25)  [unwired: 1 in]
                        n2482 = Unbundle By Name(w5566) -> ("AO"=w5567:refnum<k21>[], "E_AO"=w5568:errorcluster[])
                        n2483 = for {
                          tunnel: w5567 -> [w5576] mode=indexing
                          tunnel: w5568 -> [w5575] mode=indexing
                          tunnel: [w5574] -> w5570 mode=indexing
                          tunnel: [w5573] -> w5571 mode=indexing
                          n2484 = call <vilib>:"DAQmx Start Task.vi"("task/channels in"=w5576, "error in"=w5575) -> ("task out"=w5574:refnum<k21>, "error out"=w5573:errorcluster)  [unwired: 12 in]
                        }
                        n2485 = call "tempconfigAO_seal.vi"("command"="get") -> ("Temp Config out"=w5569:T25)  [unwired: 1 in]
                        n2486 = Bundle By Name(cluster=w5569, "AO"=w5570, "E_AO"=w5571) -> (w5572:T25)
                        n2487 = call "tempconfigAO_seal.vi"("Temp Config in"=w5572, "command"="set") -> ()  [unwired: 1 out]
                      }
                      frame #1 {
                        n2488 = call "tempconfigAI_seal.vi"("command"="get") -> ("Temp Config out"=w5578:T26)  [unwired: 1 in]
                        n2489 = Unbundle By Name(w5578) -> ("AI"=w5583:refnum<k21>, "E_AI"=w5584:errorcluster)
                        n2490 = call <vilib>:"DAQmx Start Task.vi"("task/channels in"=w5583, "error in"=w5584) -> ("task out"=w5585:refnum<k21>, "error out"=w5586:errorcluster)  [unwired: 12 in]
                        n2491 = call "tempconfigAI_seal.vi"("command"="get") -> ("Temp Config out"=w5580:T26)  [unwired: 1 in]
                        n2492 = Bundle By Name(cluster=w5580, "AI"=w5585, "E_AI"=w5586) -> (w5582:T26)
                        n2493 = call "tempconfigAI_seal.vi"("Temp Config in"=w5582, "command"="set") -> ()  [unwired: 1 out]
                      }
                    }
                  }
                  frame #3 {
                    n2494 = while {
                      tunnel: w5587 -> [w5588]
                      stop <- w5589 stop-if-true
                      n2495 = stacked-sequence {
                        seq-local: [_ _ _ w5630 _ _] -> [_ _ _ _ w5682 _]
                        seq-local: [w5591 _ _ _ _ _] -> [_ w5600 _ w5623 w5671 w5702]
                        tunnel: w5588 -> [_ _ w5608 _ w5670 _]
                        frame #0 {
                          n2496 = call "patchparameters.vi"("command"="get") -> ("Params out"=w5598:T13)  [unwired: 1 in]
                          n2497 = local read "Vholding (mV)"() -> (w5595:sgl)
                          n2498 = Unbundle By Name(w5598) -> ("Vhold (mV)"=w5594:sgl, "holdon"=w5597:bool)
                          n2499 = local read "holdon"() -> (w5596:bool)
                          n2500 = Not Equal?(x=w5595, y=w5594) -> (x != y?=w5593:bool)
                          n2501 = Not Equal?(x=w5597, y=w5596) -> (x != y?=w5592:bool)
                          n2502 = Or(x=w5593, y=w5592) -> (x .or. y?=w5591:bool)
                        }
                        frame #1 {
                          n2503 = case shown="True" w5600 {
                            frame False {
                            }
                            frame True {
                              n2504 = local read "Vholding (mV)"() -> (w5603:sgl)
                              n2505 = local read "holdon"() -> (w5601:bool)
                              n2506 = call "patchparameters.vi"("command"="get") -> ("Params out"=w5604:T13)  [unwired: 1 in]
                              n2507 = Bundle By Name(cluster=w5604, "Vhold (mV)"=w5603, "holdon"=w5601) -> (w5602:T13)
                              n2508 = call "patchparameters.vi"("Params in"=w5602, "command"="set") -> ()  [unwired: 1 out]
                            }
                          }
                        }
                        frame #2 {
                          n2509 = call "tempconfigAI_seal.vi"("command"="get") -> ("Temp Config out"=w5618:T26)  [unwired: 1 in]
                          n2510 = Unbundle By Name(w5618) -> ("AI"=w5617:refnum<k21>, "E_AI"=w5616:errorcluster)
                          n2511 = call-poly <vilib>:"DAQmx Read.vi"("task/channels in"=w5617, "number of samples per channel"=w5608, "timeout"=10.0, "error in"=w5616) -> ("task out"=w5612:refnum<k21>, "data"=w5609:i16[][], "error out"=w5621:errorcluster)  [unwired: 9 in]
                          n2512 = call "tempconfigAI_seal.vi"("command"="get") -> ("Temp Config out"=w5613:T26)  [unwired: 1 in]
                          n2513 = Bundle By Name(cluster=w5613, "AI"=w5612, "E_AI"=w5621) -> (w5620:T26)
                          n2514 = To Single Precision Float(number=w5609) -> (single precision float=w5611:sgl[][])
                          n2515 = call "tempconfigAI_seal.vi"("Temp Config in"=w5620, "command"="set") -> ()  [unwired: 1 out]
                          n2516 = call "allAI-temp.vi"("array in"=w5611, "command"=enum16{"get", "set", "clear", "append"}."set") -> ()  [unwired: 2 in, 2 out]
                        }
                        frame #3 {
                          n2517 = case shown="True" w5623 {
                            frame False {
                            }
                            frame True {
                              n2518 = call "tempconfigAO_seal.vi"("command"="get") -> ("Temp Config out"=w5659:T25)  [unwired: 1 in]
                              n2519 = Unbundle By Name(w5659) -> ("AO"=w5658:refnum<k21>[], "E_AO"=w5657:errorcluster[])
                              n2520 = call "tempconfigAI_seal.vi"("command"="get") -> ("Temp Config out"=w5646:T26)  [unwired: 1 in]
                              n2521 = Unbundle By Name(w5646) -> ("AI"=w5647:refnum<k21>, "E_AI"=w5648:errorcluster)
                              n2522 = for {
                                tunnel: w5658 -> [w5663] mode=indexing
                                tunnel: w5657 -> [w5662] mode=indexing
                                tunnel: [w5661] -> w5653 mode=indexing
                                n2523 = call <vilib>:"DAQmx Stop Task.vi"("task/channels in"=w5663, "error in"=w5662) -> ("task out"=w5664:refnum<k21>, "error out"=w5665:errorcluster)  [unwired: 12 in]
                                n2524 = call <vilib>:"DAQmx Clear Task.vi"("task in"=w5664, "error in"=w5665) -> ("error out"=w5661:errorcluster)  [unwired: 13 in]
                              }
                              n2525 = call <vilib>:"DAQmx Stop Task.vi"("task/channels in"=w5647, "error in"=w5648) -> ("task out"=w5644:refnum<k21>, "error out"=w5643:errorcluster)  [unwired: 12 in]
                              n2526 = call <vilib>:"DAQmx Clear Task.vi"("task in"=w5644, "error in"=w5643) -> ("error out"=w5642:errorcluster)  [unwired: 13 in]
                              n2527 = call "tempconfigAO_seal.vi"("command"="get") -> ("Temp Config out"=w5654:T25)  [unwired: 1 in]
                              n2528 = Bundle By Name(cluster=w5654, "E_AO"=w5653) -> (w5652:T25)
                              n2529 = call "tempconfigAI_seal.vi"("command"="get") -> ("Temp Config out"=w5650:T26)  [unwired: 1 in]
                              n2530 = Bundle By Name(cluster=w5650, "E_AI"=w5642) -> (w5641:T26)
                              n2531 = call "tempconfigAO_seal.vi"("Temp Config in"=w5652, "command"="set") -> ()  [unwired: 1 out]
                              n2532 = call "tempconfigAI_seal.vi"("Temp Config in"=w5641, "command"="set") -> ()  [unwired: 1 out]
                            }
                          }
                          n2533 = call "allAI-temp.vi"("command"=enum16{"get", "set", "clear", "append"}."get") -> ("array out"=w5627:sgl[][])  [unwired: 3 in, 1 out]
                          n2534 = call "tempconfigAI_seal.vi"("command"="get") -> ("Temp Config out"=w5639:T26)  [unwired: 1 in]
                          n2535 = Unbundle By Name(w5639) -> ("header"=w5622:dbl[])
                          n2536 = Index Array(array=w5627, index (row) #1=1 ("index (row)"), index (row) #2=0 ("index (row)")) -> (element #1=w5625:sgl[], element #2=w5624:sgl[])  [unwired: 2 in]
                          n2537 = local read "OCgain"() -> (w5632:sgl)
                          n2538 = call "Unscaledtoscaled.vi"("Unscaled Data"=w5625, "Header Information"=w5622) -> ("Array"=w5637:sgl[])  [unwired: 1 in]
                          n2539 = call "Unscaledtoscaled.vi"("Unscaled Data"=w5624, "Header Information"=w5622) -> ("Array"=w5640:sgl[])  [unwired: 1 in]
                          n2540 = Multiply(x=w5637, y=0.1) -> (x*y=w5634:dbl[])
                          n2541 = Divide(x=w5640, y=w5632) -> (x/y=w5633:sgl[])
                          n2542 = Build Array(w5634, w5633) -> (w5636:dbl[][])
                          n2543 = Multiply(x=w5636, y=1000.0) -> (x*y=w5630:dbl[][])
                          "Patch readout" <- w5630
                        }
                        frame #4 {
                          n2544 = case shown="True" w5671 {
                            tunnel: w5670 -> [_ w5683]
                            frame False {
                            }
                            frame True {
                              n2545 = call "patchparameters.vi"("command"="get") -> ("Params out"=w5687:T13)  [unwired: 1 in]
                              n2546 = Unbundle By Name(w5687) -> ("holdon"=w5686:bool, "Vhold (mV)"=w5685:sgl, "CC_icg (pA/mv)"=w5693:sgl, "CC"=w5691:bool, "VC_icg (mV/mV)"=w5692:sgl)
                              n2547 = Select(t=w5693, s=w5691, f=w5692) -> (s? t:f=w5694:sgl)
                              n2548 = To Single Precision Float(number=0.001 ("y")) -> (single precision float=w5695:sgl)
                              n2549 = Compound Arithmetic op=MULTIPLY(w5685, w5694, w5695) -> (w5689:sgl)
                              n2550 = case shown="True" w5686 {
                                tunnel: w5689 -> [_ w5700]
                                tunnel: [0.0 w5700] -> w5684
                                frame False {
                                }
                                frame True {
                                }
                              }
                              n2551 = flat-sequence {
                                tunnel: w5683 -> [w5696]
                                tunnel: w5684 -> [w5698]
                                tunnel: w5683 -> [w5697]
                                frame #0 {
                                n2552 = call "prepAI_sealtest.vi"("samples per channel"=w5696) -> ()  [unwired: 2 in]
                                }
                                frame #1 {
                                n2553 = call "prepAO_sealtest.vi"("Vhold"=w5698, "samples per channel"=w5697) -> ()  [unwired: 1 in]
                                }
                              }
                            }
                          }
                          n2554 = call "sealtestwfparams.vi"("command"="get") -> ("Params out"=w5676:T22)  [unwired: 6 in]
                          n2555 = Unbundle By Name(w5676) -> ("AO parameters"=w5677:T23)
                          n2556 = Index Array(array=w5677, index=0) -> (element=w5679:T24)
                          n2557 = Unbundle By Name(w5679) -> ("Cycles"=w5674:dbl, "Start amplitude (V)"=w5673:dbl, "Sampling frequency (Hz)"=w5672:dbl)
                          n2558 = local read "fitpoints"() -> (w5680:dbl)
                          n2559 = script code="V=data(1,:);\nI=data(2,:);\ntres=mean(V);\nspc=(nsamp./ncyc);\nV=V(spc+1:end-spc);\nI=I(spc+1:end-spc);\ndV=mean(V(V>tres))-mean(V(V<tres))\nIcyc=reshape(I,[spc ncyc-2]);\nIcyc=Icyc';\nIcyc=mean(Icyc,1);\ndIss=mean(Icyc(floor(spc*0.15):floor(spc/2)-2))-mean(Icyc(spc*0.65:spc-2))\nRm=dV*1e3/dIss;\n[maxi,ind]=max(Icyc);\nIfit=Icyc(ind+1:ind+1+points-1)-0.5*(mean(Icyc(floor(spc*0.15):floor(spc/2)-2))+mean(Icyc(spc*0.65:spc-2)))\nt=(3:points-1+3)./srate*1000;\nt=t';\nIfit=Ifit';\nc=fit(t,Ifit, 'exp1');\ncoeffs=coeffvalues(c);\nIa=coeffs(1);\nRa=dV*1e3./Ia/2;\ntau=-1./coeffs(2);\ncap=tau/Ra*1000;"("data"=w5682, "nsamp"=w5670, "ncyc"=w5674, "maxV"=w5673, "points"=w5680, "srate"=w5672) -> ("cap"=w5669:dbl, "Ra"=w5668:dbl, "Icyc"=w5667:dbl[], "Rm"=w5666:dbl)  [unwired: 1 in, 1 out]
                          n2560 = local read "set as Rp?"() -> (w5681:bool)
                          n2561 = local write "Cmembrane"(w5669) -> ()
                          n2562 = local write "Rmembrane (MOhm)"(w5666) -> ()
                          n2563 = local write "Racces (MOhm)"(w5668) -> ()
                          n2564 = case shown="True" w5681 {
                            tunnel: w5666 -> [_ w5701]
                            frame False {
                            }
                            frame True {
                              n2565 = local write "Rpipette (MOhm)"(w5701) -> ()
                            }
                          }
                          n2566 = local write "Ifit"(w5667) -> ()
                        }
                        frame #5 {
                          n2567 = local read "set as Rp?"() -> (w5703:bool)
                          n2568 = case shown="True" w5702 {
                            frame False {
                            }
                            frame True {
                              n2569 = stacked-sequence {
                                frame #0 {
                                n2570 = call "tempconfigAO_seal.vi"("command"="get") -> ("Temp Config out"=w5710:T25)  [unwired: 1 in]
                                n2571 = Unbundle By Name(w5710) -> ("AO"=w5709:refnum<k21>[], "E_AO"=w5708:errorcluster[])
                                n2572 = for {
                                tunnel: w5709 -> [w5717] mode=indexing
                                tunnel: w5708 -> [w5716] mode=indexing
                                tunnel: [w5715] -> w5706 mode=indexing
                                tunnel: [w5714] -> w5705 mode=indexing
                                n2573 = call <vilib>:"DAQmx Start Task.vi"("task/channels in"=w5717, "error in"=w5716) -> ("task out"=w5715:refnum<k21>, "error out"=w5714:errorcluster)  [unwired: 12 in]
                                }
